vi "NEW数据采集传输系统.vi"() -> ()   [LabVIEW 2016, in "数据传输系统-04.lvlib"]
uses:
  <vilib>/Utility/miscctls.llb/LVPointTypeDef.ctl
  <vilib>/Utility/error.llb/whitespace.ctl
  <vilib>/Utility/config.llb/NI_LVConfig.lvlib
  update/update.lvlib
panel:
  in  "自动更新":bool
  in  "数据补传":bool caption="确定"
  out "数据库打开失败次数":dbl
  out "与工控通信指示灯":bool
  in  "判断数据反馈":enum16{"非严格判断", "严格判断", "不判断"}(ring)
  in  "暂停上传":bool
  in  "配置表":bool caption="确定"
  in  "updateconfiguration":T1={"主机"="27.154.58.30", "用户"="update", "密码"="std23506", "远程路径"="数据传输系统\\平台数据传输系统.exe", "下载文件名"="平台数据传输系统.exe", "软件版本"=""}
  out "标题显示":string
  in  "更新":bool
  in  "系统编码选择框":string(combo)="地表水质量监测"
  in  "数据发送通道":enum16{"TCP", "VISA"}(ring)
  in  "baud rate":u32=9600 caption="波特率"
  in  "VISA resource name":refnum<visa-resource-name> caption="VISA资源名称"
  in  "实时数据发送时间间隔/min":i32=1
  in  "数据组合发送":bool
  in  "2011发送":bool
  in  "数据发送协议":enum16{"2005-212协议", "2017-212协议"}(ring)=enum."2017-212协议"
  in  "重发时间":T2(ring)
  in  "重发日期":T3(ring)
  in  "开机启动":bool
  in  "每周自动重发":bool=TRUE
  in  "确定":bool
  in  "返回":bool
  in  "PW":string
  in  "MN":string
  in  "PORT":string
  in  "IP":string
  in  "站点设备":string
  in  "站点名称":string
  out "设置超时时间/min":i32=1
  out "状态信息":T4={"1st Error to Convert "=63, "步骤 "=enum."发送数据", "元素"="实时数据", "TCP服务端掉线计数"=0, "TCP掉线时间节点"="2019/05/08 15:24:17"} {"1st Error to Convert" items=["无错误", "参数错误", "内存已满", "超出区域", "文件结束", "文件已打开", "一般文件IO错误", "未找到文件", "文件权限错误", "磁盘已满", "路径副本", "打开过多文件", "未启用", "未找到资源文件", "无法添加资源", "未找到资源", "未找到图像", "图像内存错误", "画笔不存在", "配置错误类型", "配置未找到解析段", "配置解析错误", "配置内存错误", "错误外部代码格式", "错误外部代码偏移量", "外部代码不存在", "空窗口", "销毁窗口错误", "空菜单", "打印已中止", "错误打印记录", "打印驱动程序错误", "打印时窗口错误", "打印时内存错误", "打印对话框错误", "一般打印错误", "无效设备引用句柄", "设备未找到", "设备参数错误", "设备单位错误", "无法打开设备", "设备调用已中止", "一般错误", "用户已取消", "对象ID过低", "对象ID过高", "对象不在堆中", "未知的堆", "错误DefProc ID", "DefProc不在表格中", "范围外信息", "空方法", "未知信息", "不支持管理器调用", "错误地址", "连接过程中", "连接超时", "连接过程中", "不支持网络属性", "网络错误", "正在使用的地址", "系统缺少内存", "连接已中止", "连接已拒绝", "连接未建立", "连接已建立", "连接已关闭", "初始化错误（交互应用程序管理器）", "错误事件发生", "等待无约束事件发生处理程序", "事件发生队列溢出", "错误路径", "未发出信号量", "未识别类型（交互应用程序管理器）"]}
  out "数据接收超时指示灯":bool
  out "空闲时间/s":string
  out "系统时间":string
  out "实时小时数据上传":bool
  out "系统状态改变":bool
  out "软件版本":string
  out "掉线指示":bool
  out "核查数据上传":bool
  out "配置信息":T5
  in  "参数配置":bool
  out "反控数据发送":bool
  out "读取报文显示":string
  out "发送报文显示":string
  out "心跳包":bool
  out "通信状态":bool
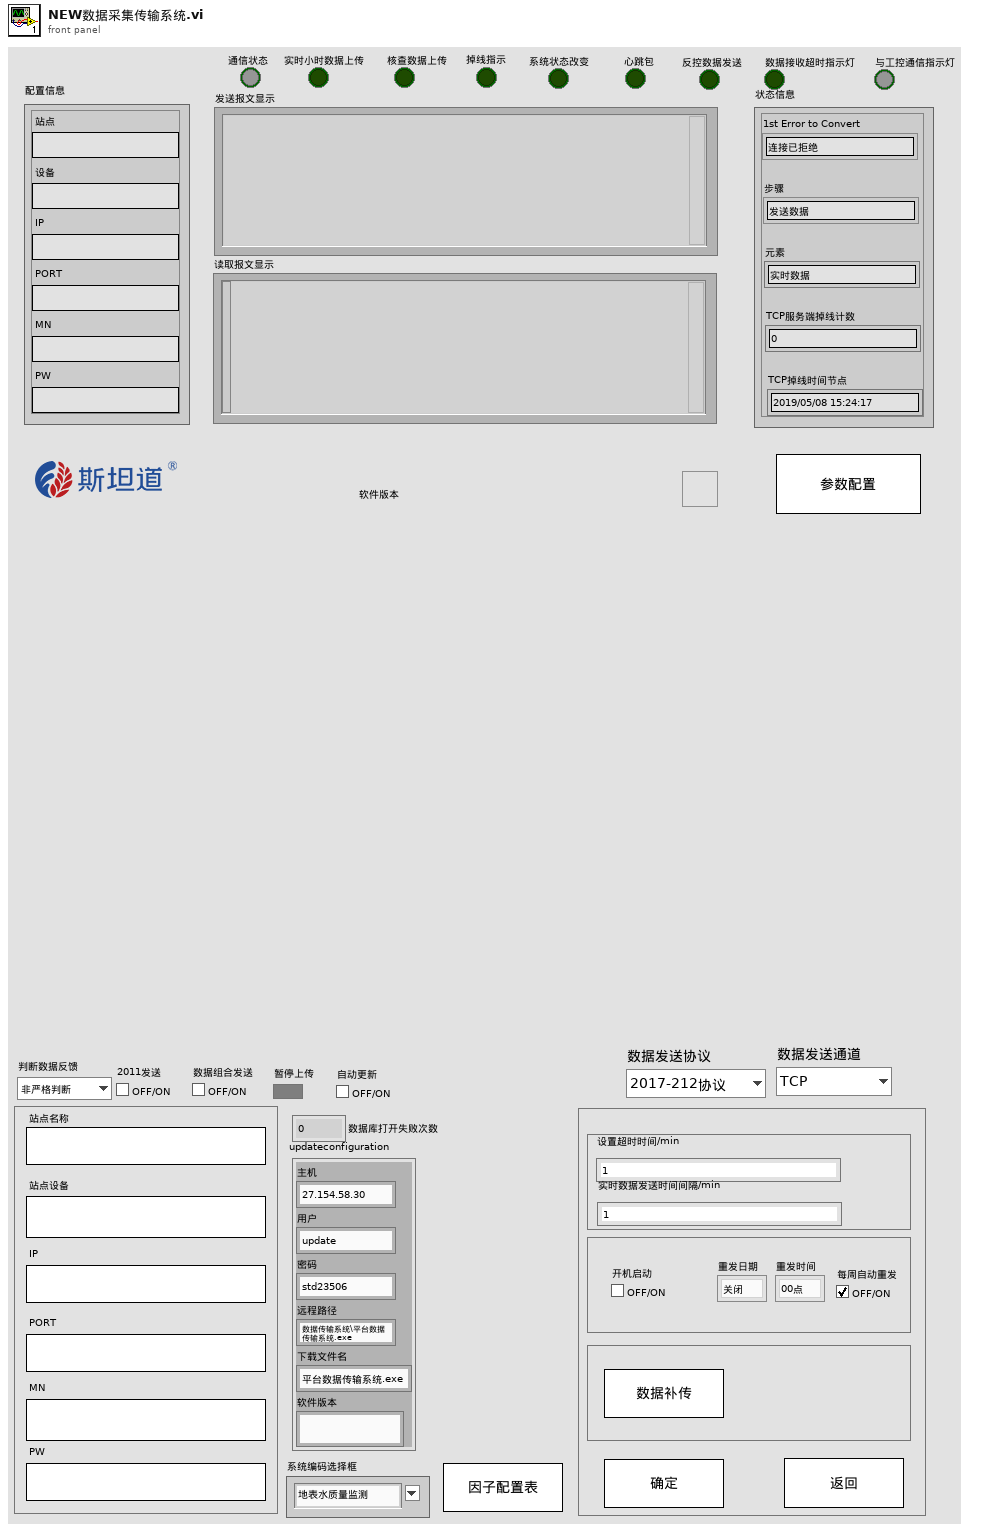
[diagram p1: front panel]
types:
  T1 = cluster{"主机":string, "用户":string, "密码":string, "远程路径":string, "下载文件名":string, "软件版本":string}
  T2 = enum16{"00点", "01点", "02点", "03点", "04点", "05点", "06点", "07点", "08点", "09点", "10点", "11点", "12点", "13点", "14点", "15点", "16点", "17点", "18点", "19点", "20点", "21点", "22点", "23点"}
  T3 = enum16{"关闭", "星期日", "星期一", "星期二", "星期三", "星期四", "星期五", "星期六"}
  T4 = cluster{"1st Error to Convert ":i32, "步骤 ":enum16{"打开连接", "发送数据", "读取数据", "数据处理", "关闭连接"}, "元素":string, "TCP服务端掉线计数":i32, "TCP掉线时间节点":string}
  T5 = cluster{"站点":string, "设备":string, "IP":string, "PORT":string, "MN":string, "PW":string}
  T6 = typedef "LVPointTypeDef.ctl" = cluster{"Horizontal":i16, "Vertical":i16}
  T7 = cluster{"setini":string, "sysini":string, "hechaini":string, "actualwrite":string, "actualread":string, "datasent":string, "反控命令信息队列":string, "反控与仪器交互":string}
  T8 = typedef "imagedata.ctl" = cluster{"image type":i32, "image depth":i32, "image":u8[], "mask":u8[], "colors":u32[], "Rectangle":cluster{"left":i16, "top":i16, "right":i16, "bottom":i16}}
  T9 = cluster{"配置表格[0]":string, "配置表格[1]":string, "配置表格[2]":string, "配置表格[3]":string, "配置表格[4]":string, "配置表格[5]":string, "配置表格[6]":string, "配置表格[7]":string, "配置表格[8]":string, "配置表格[9]":string, "配置表格[10]":string, "配置表格[11]":string, "配置表格[12]":string, "配置表格[13]":string, "配置表格[14]":string, "配置表格[15]":string, "配置表格[16]":string, "配置表格[17]":string, "配置表格[18]":string, "配置表格[19]":string, "配置表格[20]":string, "配置表格[21]":string, "配置表格[22]":string, "配置表格[23]":string, "配置表格[24]":string, "配置表格[25]":string, "配置表格[26]":string, "配置表格[27]":string, "配置表格[28]":string, "配置表格[29]":string, "配置表格[30]":string, "配置表格[31]":string, "配置表格[32]":string, "配置表格[33]":string}
  T10 = cluster{"[0]":dbl, "[1]":dbl, "[2]":dbl, "[3]":dbl, "[4]":dbl, "[5]":dbl, "[6]":dbl, "[7]":dbl, "[8]":dbl, "[9]":dbl, "[10]":dbl, "[11]":dbl, "[12]":dbl, "[13]":dbl, "[14]":dbl, "[15]":dbl, "[16]":dbl, "[17]":dbl, "[18]":dbl, "[19]":dbl, "[20]":dbl, "[21]":dbl, "[22]":dbl, "[23]":dbl, "[24]":dbl, "[25]":dbl, "[26]":dbl, "[27]":dbl, "[28]":dbl, "[29]":dbl, "[30]":dbl, "[31]":dbl, "[32]":dbl, "[33]":dbl}
  T11 = cluster{"host":string, "port":u16, "user":string, "password":string, "远端地址":string}
  T12 = typedef "NI_LVConfig.lvlib/Config Data RefNum.ctl" = refnum<k1>
  T13 = cluster{"[0]":string, "[1]":string, "[2]":string, "[3]":string, "[4]":string, "[5]":string}
  T14 = cluster{"[0]":string, "[1]":string, "[2]":string, "[3]":string, "[4]":string, "[5]":string, "[6]":string, "[7]":string}
  T15 = cluster{"[0]":string, "[1]":string, "[2]":string, "[3]":string, "[4]":string}
  T16 = cluster{"[0]":string, "[1]":string, "[2]":string, "[3]":string, "[4]":string, "[5]":string, "[6]":string, "[7]":string, "[8]":string, "[9]":string, "[10]":string, "[11]":string, "[12]":string, "[13]":string, "[14]":string}
  T17 = cluster{"[0]":string, "[1]":string, "[2]":string, "[3]":string, "[4]":string, "[5]":string, "[6]":string, "[7]":string, "[8]":string, "[9]":string, "[10]":string, "[11]":string, "[12]":string, "[13]":string, "[14]":string, "[15]":string, "[16]":string, "[17]":string, "[18]":string, "[19]":string, "[20]":string, "[21]":string, "[22]":string, "[23]":string, "[24]":string, "[25]":string, "[26]":string, "[27]":string, "[28]":string, "[29]":string, "[30]":string, "[31]":string, "[32]":string, "[33]":string}
  T18 = cluster{"[0]":string, "[1]":string, "[2]":string, "[3]":string, "[4]":string, "[5]":string, "[6]":string, "[7]":string, "[8]":string, "[9]":string, "[10]":string, "[11]":string, "[12]":string}
  T19 = typedef "whitespace.ctl" = u16
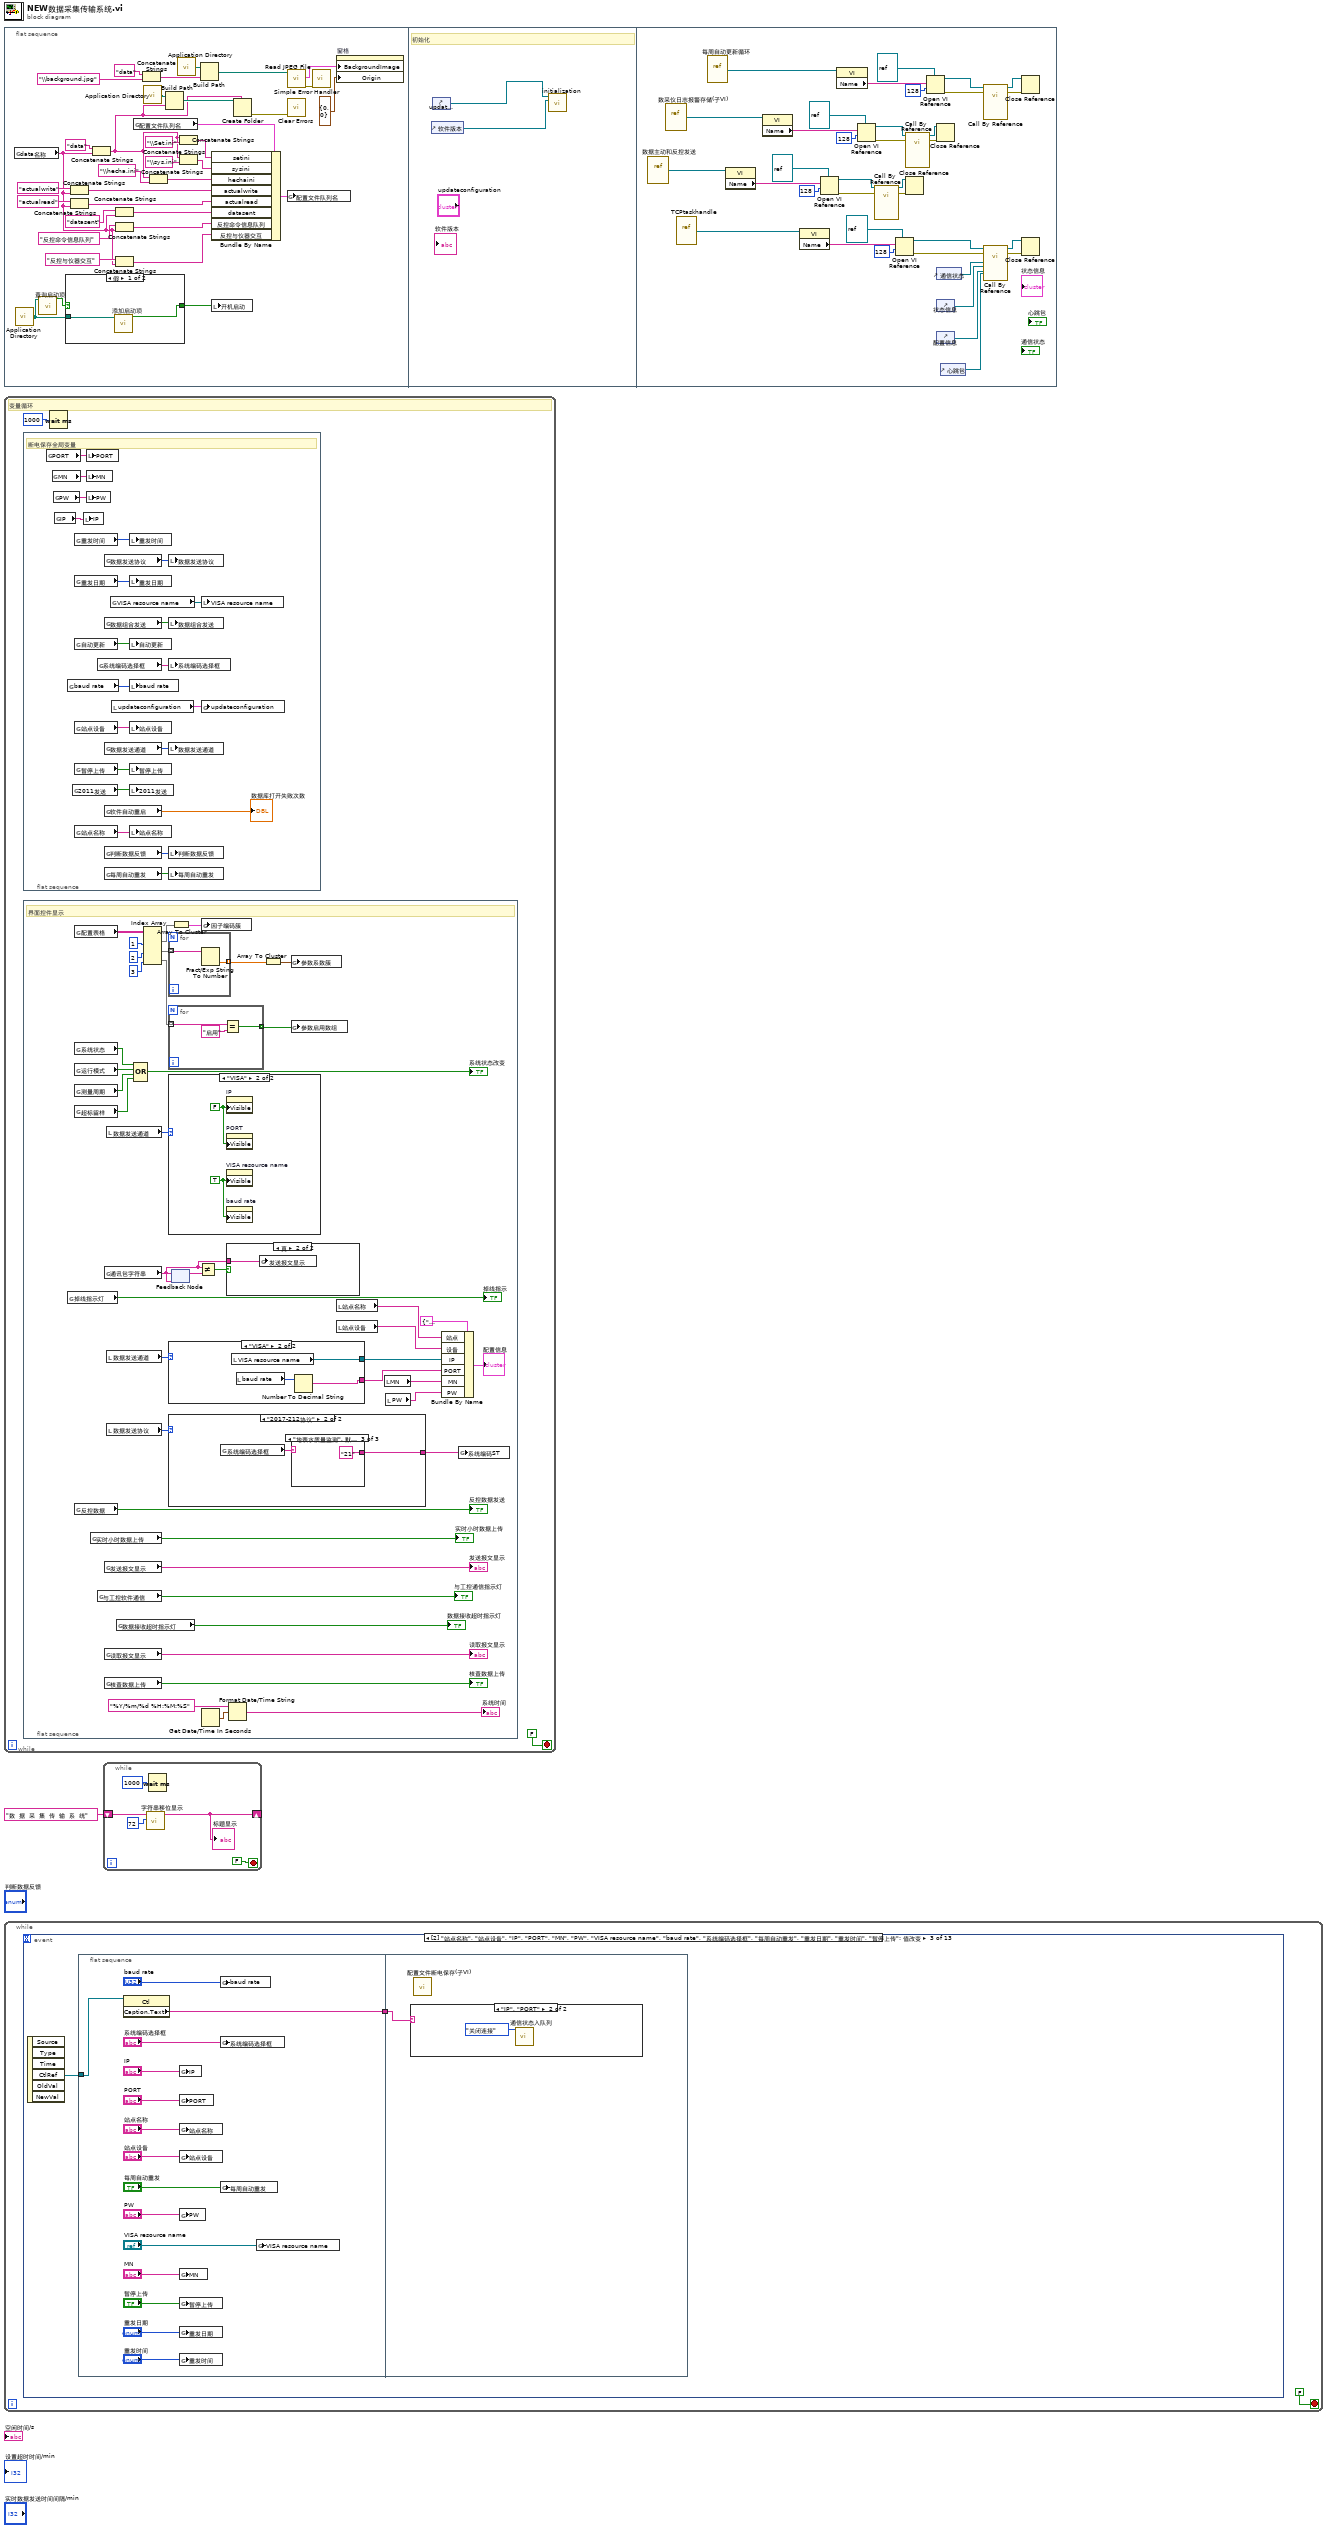
[diagram p0: block diagram]
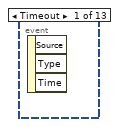
[diagram p2: hidden frame]
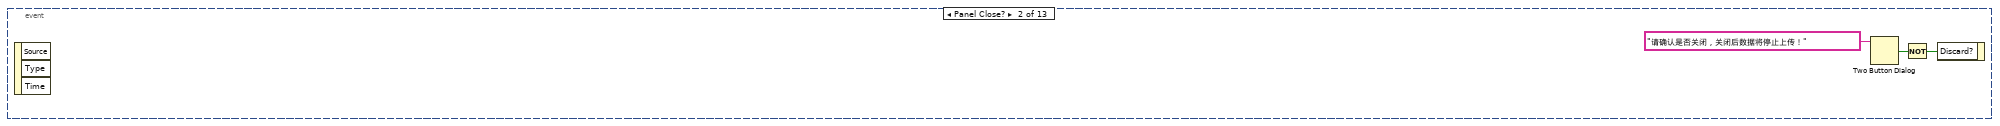
[diagram p3: hidden frame]
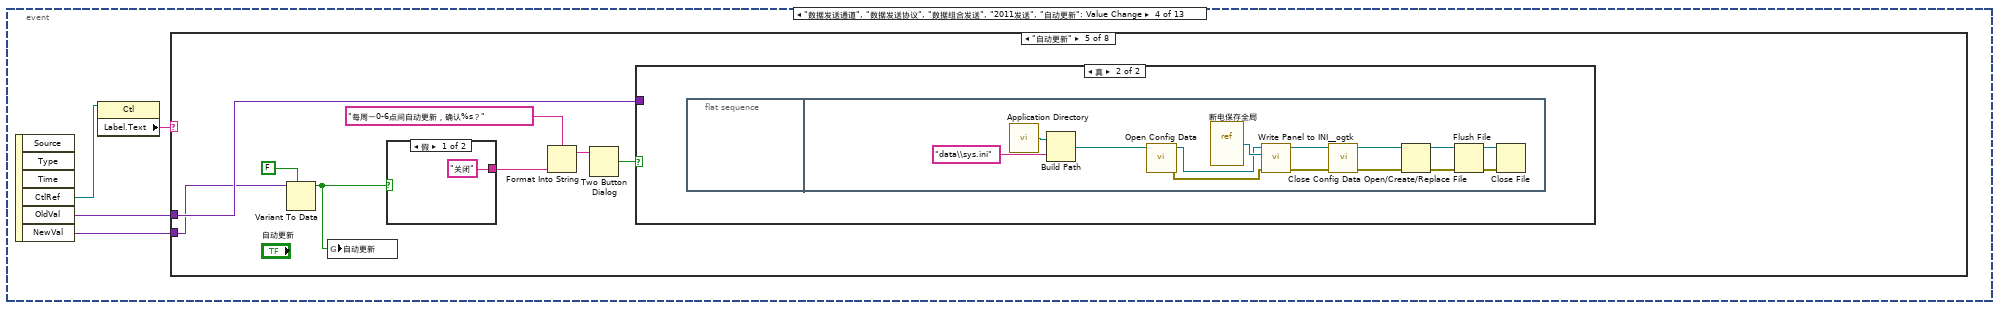
[diagram p5: hidden frame]
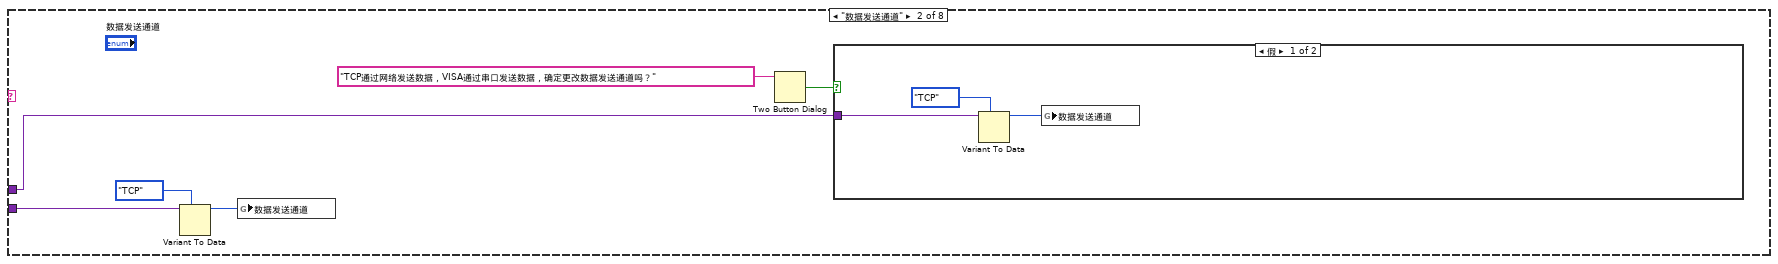
[diagram p7: hidden frame]
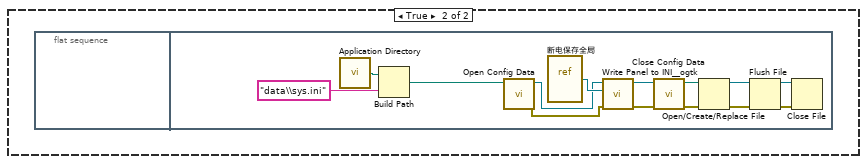
[diagram p8: hidden frame]
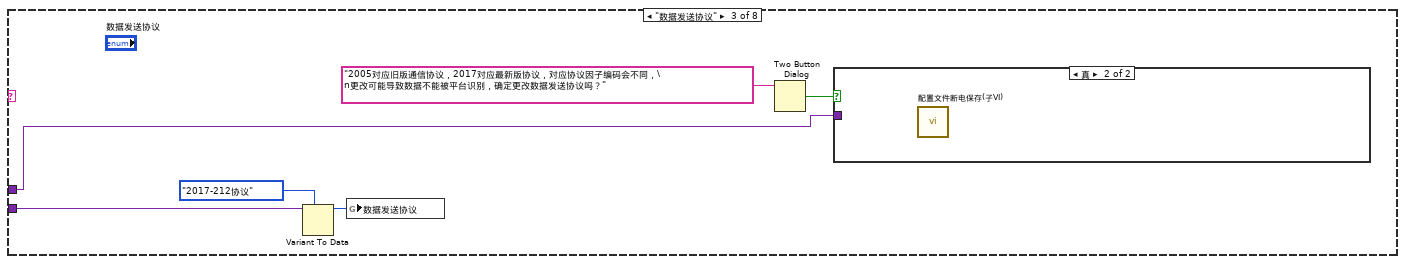
[diagram p9: hidden frame]
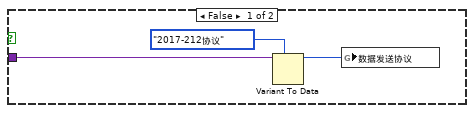
[diagram p10: hidden frame]
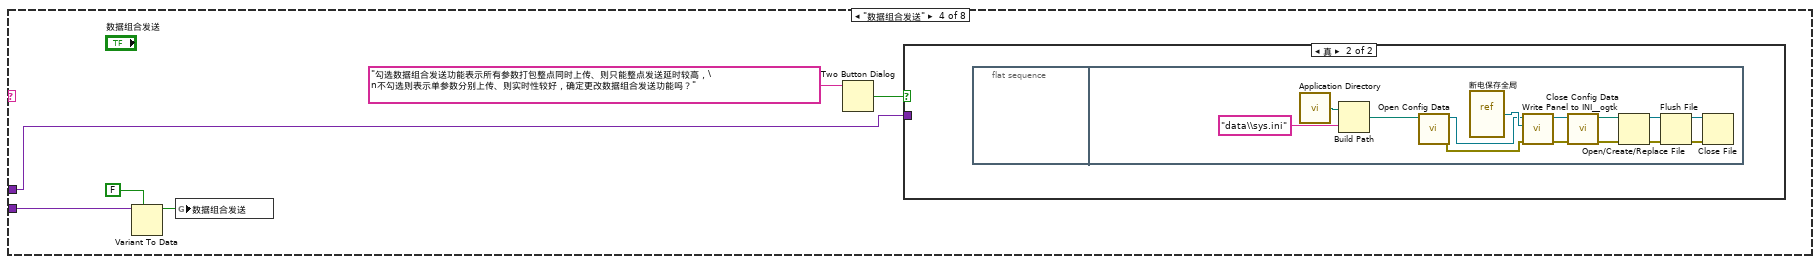
[diagram p11: hidden frame]
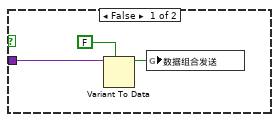
[diagram p12: hidden frame]
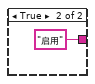
[diagram p13: hidden frame]
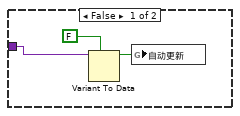
[diagram p14: hidden frame]
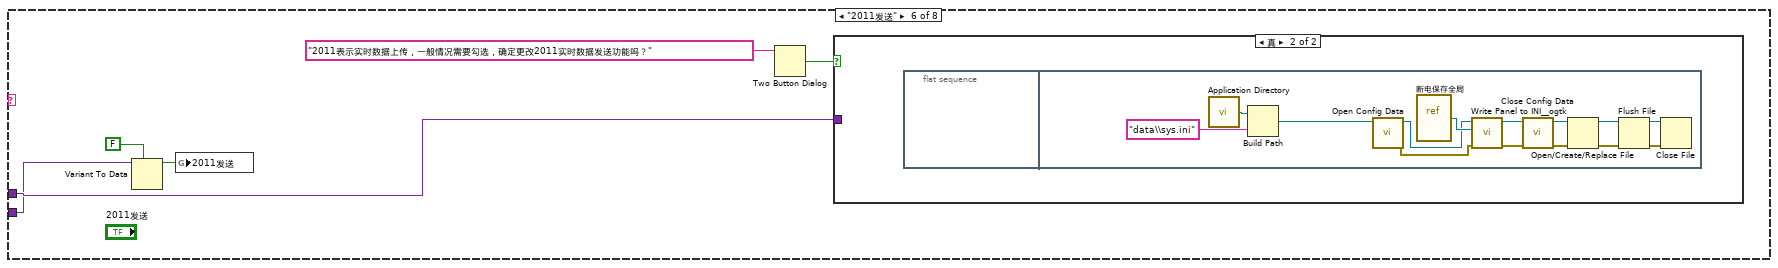
[diagram p15: hidden frame]
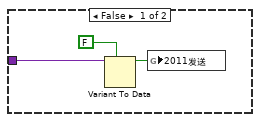
[diagram p16: hidden frame]
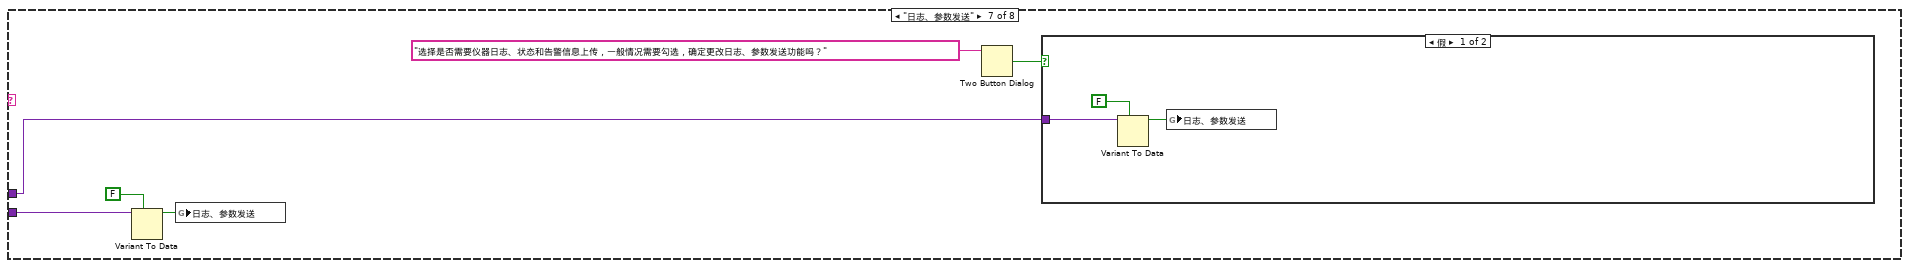
[diagram p17: hidden frame]
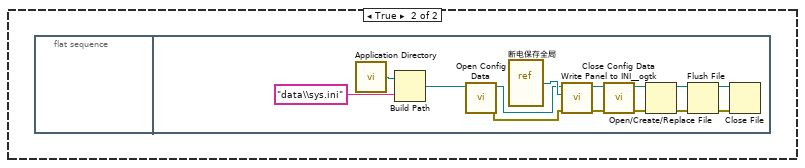
[diagram p18: hidden frame]
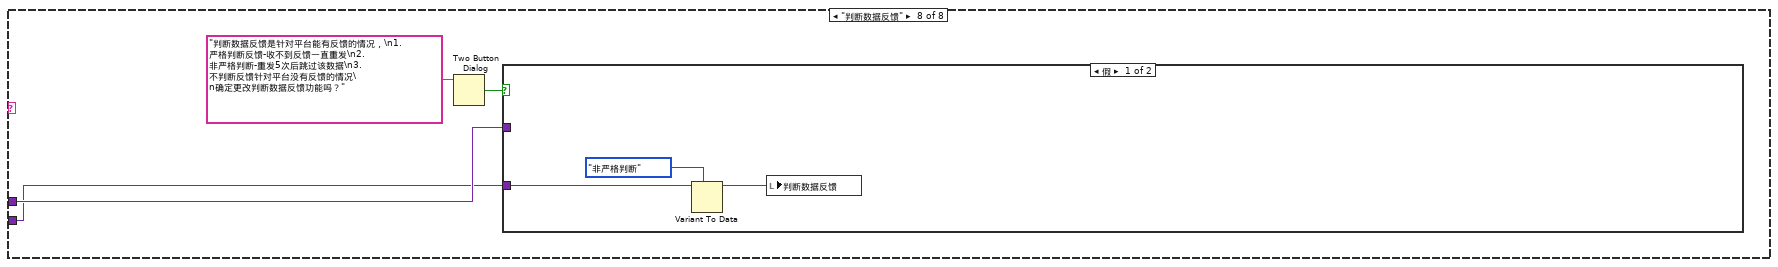
[diagram p19: hidden frame]
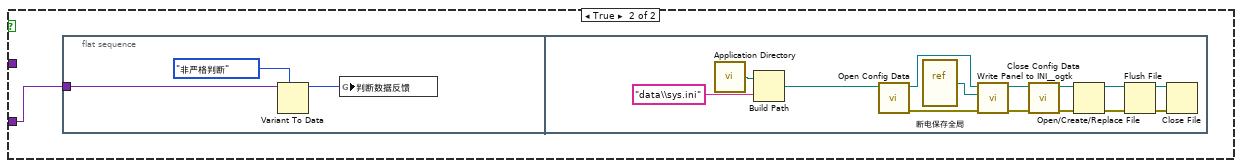
[diagram p20: hidden frame]
diagram:
  n1 = flat-sequence {
    frame #0 {
      n2 = global read "断电保存全局.vi" "data名称"() -> (w15:string)
      n3 = call <vilib>:"Application Directory.vi"() -> ("Application Directory"=w4:path)
      n4 = call "查询启动项.vi"("启动文件路径"=w4) -> ("包含启动项"=w3:bool)  [unwired: 9 in, 1 out]
      n5 = case shown="假" w3 {
        selector: w3 -> [_ w39]
        tunnel: w4 -> [w38 _]
        tunnel: [w37 w39] -> w2
        frame False {
          n6 = call "添加启动项.vi"("启动文件路径"=w38) -> ("添加成功标记"=w37:bool)  [unwired: 9 in, 1 out]
        }
        frame True {
        }
      }
      n7 = Concatenate Strings("actualwrite" ("名称（未命名）"), w15) -> (w24:string)
      n8 = Concatenate Strings("actualread" ("名称（未命名）"), w15) -> (w22:string)
      n9 = Concatenate Strings("data" ("对话框窗口（创建文件夹）"), w15) -> (w29:string)
      n10 = Concatenate Strings("datasent" ("名称（未命名）"), w15) -> (w20:string)
      n11 = Concatenate Strings("反控命令信息队列" ("名称（未命名）"), w15) -> (w13:string)
      n12 = Concatenate Strings("反控与仪器交互" ("名称（未命名）"), w15) -> (w14:string)
      n13 = global read "断电保存全局.vi" "配置文件队列名"() -> (w19:T7)
      n14 = Concatenate Strings("data" ("名称或相对路径"), "\\background.jpg" ("名称或相对路径")) -> (w10:string)
      n15 = call <vilib>:"Application Directory.vi"() -> ("Application Directory"=w35:path)
      n16 = Concatenate Strings(w29, "\\hecha.ini" ("名称或相对路径")) -> (w27:string)
      n17 = Build Path(base path=w35, name or relative path=w29) -> (appended path=w34:path)
      n18 = call <vilib>:"Application Directory.vi"() -> ("Application Directory"=w5:path)
      n19 = Concatenate Strings(w29, "\\Set.ini" ("名称或相对路径")) -> (w31:string)
      n20 = Concatenate Strings(w29, "\\sys.ini" ("名称或相对路径")) -> (w28:string)
      n21 = Build Path(base path=w5, name or relative path=w10) -> (appended path=w6:path)
      n22 = Bundle By Name(cluster=w19, "setini"=w31, "sysini"=w28, "hechaini"=w27, "actualwrite"=w24, "actualread"=w22, "datasent"=w20, "反控命令信息队列"=w13, "反控与仪器交互"=w14) -> (w18:T7)
      n23 = local write "开机启动"(w2) -> ()
      n24 = Create Folder(prompt (Create Folder)=w29, path (use dialog)=w34) -> (error out=w33:errorcluster)  [unwired: 1 in, 2 out]
      n25 = call <vilib>:"Read JPEG File.vi"("path to JPEG file"=w6) -> ("error out"=w8:errorcluster, "image data"=w7:T8)  [unwired: 8 in, 1 out]
      n26 = call <vilib>:"Clear Errors.vi"("error in (no error)"=w33) -> ()  [unwired: 5 in, 2 out]
      n27 = global write "断电保存全局.vi" "配置文件队列名"(w18) -> ()
      n28 = call <vilib>:"Simple Error Handler.vi"("error in (no error)"=w8) -> ()  [unwired: 4 in, 5 out]
      n29 = property on="窗格" class="Pane"("BackgroundImage"=w7, "Origin"=T6 {"Horizontal"=0, "Vertical"=0} ("原点")) -> ()  [unwired: 2 in, 2 out]
    }
    frame #1 {
      # "初始化"
      n30 = control-ref of="软件版本"() -> (w40:refnum<vi>)
      n31 = control-ref of="updateconfiguration"() -> (w41:refnum<vi>)
      n32 = call "initialization.vi"("软件版本"=w40, "updateconfiguration"=w41) -> ()  [unwired: 9 in]
    }
    frame #2 {
      n33 = vi-ref "数据主动和反控发送.vi"() -> (w69:refnum<vi>)
      n34 = vi-ref "数采仪日志报警存储(子VI).vi"() -> (w70:refnum<vi>)
      n35 = vi-ref "TCPtaskhandle.vi"() -> (w46:refnum<vi>)
      n36 = vi-ref "每周自动更新循环.vi"() -> (w61:refnum<vi>)
      n37 = property class="VI"(reference=w69) -> ("Name"=w68:string)  [unwired: 1 in, 2 out]
      n38 = property class="VI"(reference=w70) -> ("Name"=w77:string)  [unwired: 1 in, 2 out]
      n39 = property class="VI"(reference=w46) -> ("Name"=w53:string)  [unwired: 1 in, 2 out]
      n40 = Open VI Reference(type specifier VI Refnum (for type only)=refnum<vi> refnum, vi path=w68, options=128 ("选项")) -> (vi reference=w66:refnum<vi>, error out=w64:errorcluster)  [unwired: 3 in]
      n41 = property class="VI"(reference=w61) -> ("Name"=w54:string)  [unwired: 1 in, 2 out]
      n42 = Open VI Reference(type specifier VI Refnum (for type only)=refnum<vi> refnum, vi path=w77, options=128 ("选项")) -> (vi reference=w75:refnum<vi>, error out=w73:errorcluster)  [unwired: 3 in]
      n43 = call-by-ref "?"(reference=w66, error in=w64) -> (reference out=w62:refnum<vi>, error out=w63:errorcluster)  [unwired: 12 in]
      n44 = Open VI Reference(type specifier VI Refnum (for type only)=refnum<vi> refnum, vi path=w53, options=128 ("选项")) -> (vi reference=w51:refnum<vi>, error out=w49:errorcluster)  [unwired: 3 in]
      n45 = call-by-ref "?"(reference=w75, error in=w73) -> (reference out=w71:refnum<vi>, error out=w72:errorcluster)  [unwired: 12 in]
      n46 = Close Reference(reference=w62, error in (no error)=w63) -> ()  [unwired: 1 out]
      n47 = Open VI Reference(type specifier VI Refnum (for type only)=refnum<vi> refnum, vi path=w54, options=128 ("选项")) -> (vi reference=w56:refnum<vi>, error out=w58:errorcluster)  [unwired: 3 in]
      n48 = Close Reference(reference=w71, error in (no error)=w72) -> ()  [unwired: 1 out]
      n49 = control-ref of="通信状态"() -> (w45:refnum<vi>)
      n50 = control-ref of="状态信息"() -> (w44:refnum<vi>)
      n51 = control-ref of="配置信息"() -> (w43:refnum<vi>)
      n52 = control-ref of="心跳包"() -> (w42:refnum<vi>)
      n53 = call-by-ref "?"(reference=w56, error in=w58) -> (reference out=w60:refnum<vi>, error out=w59:errorcluster)  [unwired: 12 in]
      n54 = call-by-ref "?"(reference=w51, error in=w49, "心跳包"=w42, "配置信息"=w43, "状态信息"=w44, "通信状态"=w45) -> (reference out=w47:refnum<vi>, error out=w48:errorcluster)  [unwired: 8 in]
      n55 = Close Reference(reference=w60, error in (no error)=w59) -> ()  [unwired: 1 out]
      n56 = Close Reference(reference=w47, error in (no error)=w48) -> ()  [unwired: 1 out]
    }
  }
  n57 = while {
    stop <- FALSE stop-if-true
    # "变量循环"
    n58 = flat-sequence {
      frame #0 {
        # "断电保存全局变量"
        n59 = global read "断电保存全局.vi" "PORT"() -> (w164:string)
        n60 = global read "断电保存全局.vi" "MN"() -> (w163:string)
        n61 = global read "断电保存全局.vi" "PW"() -> (w162:string)
        n62 = global read "断电保存全局.vi" "IP"() -> (w165:string)
        n63 = global read "断电保存全局.vi" "baud rate"() -> (w160:u32)
        n64 = global read "断电保存全局.vi" "2011发送"() -> (w156:bool)
        n65 = global read "断电保存全局.vi" "重发时间"() -> (w151:T2)
        n66 = global read "断电保存全局.vi" "重发日期"() -> (w158:T3)
        n67 = global read "断电保存全局.vi" "自动更新"() -> (w147:bool)
        n68 = global read "断电保存全局.vi" "站点设备"() -> (w166:string)
        n69 = global read "断电保存全局.vi" "暂停上传"() -> (w149:bool)
        n70 = global read "断电保存全局.vi" "站点名称"() -> (w167:string)
        n71 = local write "IP"(w165) -> ()
        n72 = local write "PORT"(w164) -> ()
        n73 = local write "MN"(w163) -> ()
        n74 = local write "PW"(w162) -> ()
        n75 = global read "断电保存全局.vi" "系统编码选择框"() -> (w152:string)
        n76 = global read "断电保存全局.vi" "数据发送协议"() -> (w154:enum16{"2005-212协议", "2017-212协议"})
        n77 = global read "断电保存全局.vi" "数据组合发送"() -> (w155:bool)
        n78 = global read "断电保存全局.vi" "数据发送通道"() -> (w153:enum16{"TCP", "VISA"})
        n79 = global read "全局1.vi" "软件自动重启"() -> (→"数据库打开失败次数":dbl)
        n80 = global read "断电保存全局.vi" "判断数据反馈"() -> (w157:enum16{"非严格判断", "严格判断", "不判断"})
        n81 = global read "断电保存全局.vi" "每周自动重发"() -> (w159:bool)
        n82 = global read "断电保存全局.vi" "VISA resource name"() -> (w161:refnum<visa-resource-name>)
        n83 = local read "updateconfiguration"() -> (w150:T1)
        n84 = local write "重发时间"(w151) -> ()
        n85 = local write "重发日期"(w158) -> ()
        n86 = local write "自动更新"(w147) -> ()
        n87 = local write "baud rate"(w160) -> ()
        n88 = local write "站点设备"(w166) -> ()
        n89 = local write "暂停上传"(w149) -> ()
        n90 = local write "2011发送"(w156) -> ()
        n91 = local write "站点名称"(w167) -> ()
        n92 = local write "数据发送协议"(w154) -> ()
        n93 = local write "数据组合发送"(w155) -> ()
        n94 = local write "系统编码选择框"(w152) -> ()
        n95 = local write "数据发送通道"(w153) -> ()
        n96 = local write "判断数据反馈"(w157) -> ()
        n97 = local write "每周自动重发"(w159) -> ()
        n98 = local write "VISA resource name"(w161) -> ()
        n99 = global write "update全局.vi" "updateconfiguration"(w150) -> ()
      }
    }
    n100 = flat-sequence {
      frame #0 {
        # "界面控件显示"
        n101 = global read "全局 数据发送重叠.vi" "掉线指示灯"() -> (→"掉线指示":bool)
        n102 = global read "断电保存全局.vi" "配置表格"() -> (w90:string[][])
        n103 = global read "全局1.vi" "系统状态"() -> (w92:bool)
        n104 = global read "全局1.vi" "运行模式"() -> (w93:bool)
        n105 = global read "全局1.vi" "测量周期"() -> (w94:bool)
        n106 = global read "全局1.vi" "超标留样"() -> (w95:bool)
        n107 = global read "全局1.vi" "反控数据"() -> (→"反控数据发送":bool)
        n108 = global read "全局1.vi" "实时小时数据上传"() -> (→"实时小时数据上传":bool)
        n109 = global read "全局1.vi" "与工控软件通信"() -> (→"与工控通信指示灯":bool)
        n110 = global read "全局1.vi" "通讯包字符串"() -> (w102:string)
        n111 = global read "全局1.vi" "发送报文显示"() -> (→"发送报文显示":string)
        n112 = global read "全局1.vi" "读取报文显示"() -> (→"读取报文显示":string)
        n113 = global read "全局1.vi" "核查数据上传"() -> (→"核查数据上传":bool)
        n114 = local read "数据发送通道"() -> (w100:enum16{"TCP", "VISA"})
        n115 = local read "数据发送通道"() -> (w121:enum16{"TCP", "VISA"})
        n116 = local read "数据发送协议"() -> (w110:enum16{"2005-212协议", "2017-212协议"})
        n117 = global read "全局 数据发送重叠.vi" "数据接收超时指示灯"() -> (→"数据接收超时指示灯":bool)
        n118 = Compound Arithmetic op=OR ("复合运算")(w92, w93, w94, w95) -> (→"系统状态改变":bool)
        n119 = Index Array(array=w90, index (col) #1=1 ("禁用的索引 (列)"), index (col) #2=2 ("索引 (列)"), index (col) #3=3 ("索引 (列)")) -> (element #1=w88:string[], element #2=w82:string[], element #3=w84:string[])  [unwired: 3 in]
        n120 = for {
          tunnel: w82 -> [w123] mode=indexing
          tunnel: [w122] -> w81 mode=indexing
          n121 = Fract/Exp String To Number(string=w123) -> (number=w122:dbl)  [unwired: 3 in, 1 out]
        }
        n122 = for {
          tunnel: w84 -> [w126] mode=indexing
          tunnel: [w124] -> w83 mode=indexing
          n123 = Equal?(x=w126, y="启用") -> (x = y?=w124:bool)
        }
        n124 = case shown="\"VISA\"" w100 {
          frame "TCP", Default {
            w127 = TRUE ("可见")
            w128 = FALSE ("可见")
            n125 = property on="IP" class="Str"("Visible"=w127) -> ()  [unwired: 2 in, 2 out]
            n126 = property on="PORT" class="Str"("Visible"=w127) -> ()  [unwired: 2 in, 2 out]
            n127 = property on="VISA resource name" class="VISAName"("Visible"=w128) -> ()  [unwired: 2 in, 2 out]
            n128 = property on="baud rate" class="DigNum (严格)"("Visible"=w128) -> ()  [unwired: 2 in, 2 out]
          }
          frame "VISA" {
            w129 = FALSE ("可见")
            w130 = TRUE ("可见")
            n129 = property on="IP" class="Str"("Visible"=w129) -> ()  [unwired: 2 in, 2 out]
            n130 = property on="PORT" class="Str"("Visible"=w129) -> ()  [unwired: 2 in, 2 out]
            n131 = property on="VISA resource name" class="VISAName"("Visible"=w130) -> ()  [unwired: 2 in, 2 out]
            n132 = property on="baud rate" class="DigNum (严格)"("Visible"=w130) -> ()  [unwired: 2 in, 2 out]
          }
        }
        n133 = case shown="\"VISA\"" w121 {
          tunnel: [w143 w146] -> w118
          tunnel: [w142 w144] -> w115
          frame "TCP", Default {
            n134 = local read "PORT"() -> (w142:string)
            n135 = local read "IP"() -> (w143:string)
          }
          frame "VISA" {
            n136 = local read "VISA resource name"() -> (w146:refnum<visa-resource-name>)
            n137 = local read "baud rate"() -> (w145:u32)
            n138 = Number To Decimal String(number=w145) -> (decimal integer string=w144:string)  [unwired: 1 in]
          }
        }
        n139 = case shown="\"2017-212协议\"" w110 {
          tunnel: [w132 w137] -> w109
          frame "2005-212协议", Default {
            n140 = global read "断电保存全局.vi" "系统编码选择框"() -> (w133:string)
            n141 = case shown="\"地表水体污染源\"" w133 {
              tunnel: ["52" ("设备编码MN") "32" ("设备编码MN") "21" ("设备编码MN")] -> w132
              frame "污水排放过程监测" {
              }
              frame "地表水体污染源" {
              }
              frame "地表水质量监测", Default {
              }
            }
          }
          frame "2017-212协议" {
            n142 = global read "断电保存全局.vi" "系统编码选择框"() -> (w138:string)
            n143 = case shown="\"地表水质量监测\", 默认" w138 {
              tunnel: ["52" ("设备编码MN") "32" ("设备编码MN") "21" ("设备编码MN")] -> w137
              frame "污水排放过程监测" {
              }
              frame "地表水体污染源" {
              }
              frame "地表水质量监测", Default {
              }
            }
          }
        }
        n144 = feedback #1(w102) -> (w103:string)
        n145 = feedback-in #1(w102) -> ()
        n146 = Array To Cluster(array=w88) -> (cluster=w91:T9)
        n147 = Not Equal?(x=w102, y=w103) -> (x != y?=w101:bool)
        n148 = global write "断电保存全局.vi" "因子编码簇"(w91) -> ()
        n149 = Get Date/Time In Seconds() -> (seconds since 1Jan1904=w111:timestamp)
        n150 = case shown="真" w101 {
          tunnel: w102 -> [_ w131]
          frame False {
          }
          frame True {
            n151 = global write "全局1.vi" "发送报文显示"(w131) -> ()
          }
        }
        n152 = Format Date/Time String(time format string (%c)="%Y/%m/%d %H:%M:%S" ("时间格式字符串(%c)"), seconds (now)=w111) -> (date/time string=→"系统时间":string)  [unwired: 1 in]
        n153 = Array To Cluster(array=w81) -> (cluster=w85:T10)
        n154 = global write "断电保存全局.vi" "参数系数簇"(w85) -> ()
        n155 = global write "断电保存全局.vi" "参数启用数组"(w83) -> ()
        n156 = local read "站点名称"() -> (w117:string)
        n157 = local read "站点设备"() -> (w116:string)
        n158 = local read "MN"() -> (w114:string)
        n159 = local read "PW"() -> (w113:string)
        n160 = Bundle By Name(cluster=T5 {"站点"="", "设备"="", "IP"="", "PORT"="", "MN"="", "PW"=""} ("配置信息"), "站点"=w117, "设备"=w116, "IP"=w118, "PORT"=w115, "MN"=w114, "PW"=w113) -> (→"配置信息":T5)
        n161 = global write "全局1.vi" "系统编码ST"(w109) -> ()
      }
    }
    n162 = Wait (ms)(milliseconds to wait=u32 1000 ("等待时间（毫秒）")) -> ()  [unwired: 1 out]
  }
  n163 = while {
    stop <- FALSE stop-if-true
    n164 = event shown="[2] \"站点名称\", \"站点设备\", \"IP\", \"PORT\", \"MN\", \"PW\", \"VISA resource name\", \"baud rate\", \"系统编码选择框\", \"每周自动重发\", \"重发日期\", \"重发时间\", \"暂停上传\": 值改变" {
      selector: _ -> [_ _ _ _ _ _ _ _ _ _ _ _ _]
      dyn-events: _ -> [_ _ _ _ _ _ _ _ _ _ _ _ _]
      timeout: _ -> [_ _ _ _ _ _ _ _ _ _ _ _ _]
      event Timeout {
        n165 = event-data() -> ()  [unwired: 1 in, 3 out]
      }
      event Panel Close? {
        n166 = event-data() -> ()  [unwired: 1 in, 3 out]
        n167 = Two Button Dialog(message="请确认是否关闭，关闭后数据将停止上传！" ("消息")) -> (T button?=w171:bool)  [unwired: 2 in]
        n168 = Not(x=w171) -> (.not. x?=w170:bool)
        n169 = event-data("Discard?"=w170) -> ()  [unwired: 1 in, 1 out]
      }
      event "站点名称", "站点设备", "IP", "PORT", "MN", "PW", "VISA resource name", "baud rate", "系统编码选择框", "每周自动重发", "重发日期", "重发时间", "暂停上传": Value Change {
        n170 = event-data() -> ("CtlRef"=w173:refnum<vi>)  [unwired: 1 in, 5 out]
        n171 = flat-sequence {
          tunnel: w173 -> [w175]
          tunnel: [w174] -> w172
          tunnel: w172 -> [w189]
          frame #0 {
            n172 = property class="Ctl"(reference=w175) -> ("Caption.Text"=w174:string)  [unwired: 1 in, 2 out]
            n173 = global write "断电保存全局.vi" "IP"("IP") -> ()
            n174 = global write "断电保存全局.vi" "PORT"("PORT") -> ()
            n175 = global write "断电保存全局.vi" "站点名称"("站点名称") -> ()
            n176 = global write "断电保存全局.vi" "站点设备"("站点设备") -> ()
            n177 = global write "断电保存全局.vi" "PW"("PW") -> ()
            n178 = global write "断电保存全局.vi" "MN"("MN") -> ()
            n179 = global write "断电保存全局.vi" "暂停上传"("暂停上传") -> ()
            n180 = global write "断电保存全局.vi" "重发日期"("重发日期") -> ()
            n181 = global write "断电保存全局.vi" "重发时间"("重发时间") -> ()
            n182 = global write "断电保存全局.vi" "baud rate"("baud rate") -> ()
            n183 = global write "断电保存全局.vi" "系统编码选择框"("系统编码选择框") -> ()
            n184 = global write "断电保存全局.vi" "每周自动重发"("每周自动重发") -> ()
            n185 = global write "断电保存全局.vi" "VISA resource name"("VISA resource name") -> ()
          }
          frame #1 {
            n186 = case shown="\"IP\", \"PORT\"" w189 {
              frame "假", Default {
              }
              frame "IP", "PORT" {
                n187 = call "通信状态入队列.vi"("枚举"=enum16{"打开连接", "发送数据", "读取数据", "数据处理", "关闭连接"}."关闭连接") -> ()  [unwired: 10 in, 1 out]
              }
            }
            n188 = call "配置文件断电保存(子VI).vi"() -> ()  [unwired: 12 in]
          }
        }
      }
      event "数据发送通道", "数据发送协议", "数据组合发送", "2011发送", "自动更新": Value Change {
        n189 = event-data() -> ("CtlRef"=w194:refnum<vi>, "OldVal"=w192:variant, "NewVal"=w191:variant)  [unwired: 1 in, 3 out]
        n190 = property class="Ctl"(reference=w194) -> ("Label.Text"=w193:string)  [unwired: 1 in, 2 out]
        n191 = case shown="\"自动更新\"" w193 {
          tunnel: w192 -> [_ w198 w221 w230 w256 w280 w303 w324]
          tunnel: w191 -> [_ w195 w218 w227 w254 w277 w300 w323]
          frame "假", Default {
          }
          frame "数据发送通道" {
            n192 = Variant To Data(type=enum16{"TCP", "VISA"}."TCP" ("数据发送通道"), Variant=w195) -> (data=w196:enum16{"TCP", "VISA"})  [unwired: 1 in, 1 out]
            n193 = global write "断电保存全局.vi" "数据发送通道"(w196) -> ()
            n194 = Two Button Dialog(message="TCP通过网络发送数据，VISA通过串口发送数据，确定更改数据发送通道吗？" ("消息")) -> (T button?=w199:bool)  [unwired: 2 in]
            n195 = case shown="假" w199 {
              tunnel: w198 -> [w202 _]
              frame False {
                n196 = Variant To Data(type=enum16{"TCP", "VISA"}."TCP" ("数据发送通道"), Variant=w202) -> (data=w201:enum16{"TCP", "VISA"})  [unwired: 1 in, 1 out]
                n197 = global write "断电保存全局.vi" "数据发送通道"(w201) -> ()
              }
              frame True {
                n198 = flat-sequence {
                  frame #0 {
                  }
                  frame #1 {
                    n199 = call <vilib>:"Application Directory.vi"() -> ("Application Directory"=w204:path)
                    n200 = Build Path(base path=w204, name or relative path="data\\sys.ini" ("名称或相对路径")) -> (appended path=w206:path)
                    n201 = call <vilib>:"Open Config Data.vi"("configuration file path"=w206) -> ("error out"=w210:errorcluster, "refnum"=w207:T12)  [unwired: 8 in, 1 out]
                    n202 = vi-ref "断电保存全局.vi"() -> (w208:refnum<vi>)
                    n203 = call <userlib>:"Write Panel to INI__ogtk.vi"("error in (no error)"=w210, "VI ref"=w208, "refnum"=w207) -> ("error out"=w211:errorcluster, "refnum out"=w209:T12)  [unwired: 7 in]
                    n204 = call <vilib>:"Close Config Data.vi"("error in (no error)"=w211, "refnum"=w209) -> ("error out"=w216:errorcluster, "file path"=w217:path)  [unwired: 8 in]
                    n205 = Open/Create/Replace File(file path (use dialog)=w217, error in=w216) -> (refnum out=w213:refnum<file>, error out=w212:errorcluster)  [unwired: 4 in, 1 out]
                    n206 = Flush File(refnum=w213, error in=w212) -> (refnum out=w214:refnum<file>, error out=w215:errorcluster)
                    n207 = Close File(refnum=w214, error in=w215) -> ()  [unwired: 2 out]
                  }
                }
              }
            }
          }
          frame "数据发送协议" {
            n208 = Variant To Data(type=enum16{"2005-212协议", "2017-212协议"}."2017-212协议" ("数据"), Variant=w218) -> (data=w219:enum16{"2005-212协议", "2017-212协议"})  [unwired: 1 in, 1 out]
            n209 = global write "断电保存全局.vi" "数据发送协议"(w219) -> ()
            n210 = Two Button Dialog(message="2005对应旧版通信协议，2017对应最新版协议，对应协议因子编码会不同，\n更改可能导致数据不能被平台识别，确定更改数据发送协议吗？" ("消息")) -> (T button?=w222:bool)  [unwired: 2 in]
            n211 = case shown="真" w222 {
              tunnel: w221 -> [w226 _]
              frame False {
                n212 = Variant To Data(type=enum16{"2005-212协议", "2017-212协议"}."2017-212协议" ("数据"), Variant=w226) -> (data=w224:enum16{"2005-212协议", "2017-212协议"})  [unwired: 1 in, 1 out]
                n213 = global write "断电保存全局.vi" "数据发送协议"(w224) -> ()
              }
              frame True {
                n214 = call "配置文件断电保存(子VI).vi"() -> ()  [unwired: 12 in]
              }
            }
          }
          frame "数据组合发送" {
            n215 = Variant To Data(type=FALSE, Variant=w227) -> (data=w228:bool)  [unwired: 1 in, 1 out]
            n216 = global write "断电保存全局.vi" "数据组合发送"(w228) -> ()
            n217 = Two Button Dialog(message="勾选数据组合发送功能表示所有参数打包整点同时上传、则只能整点发送延时较高，\n不勾选则表示单参数分别上传、则实时性较好，确定更改数据组合发送功能吗？" ("消息")) -> (T button?=w231:bool)  [unwired: 2 in]
            n218 = case shown="真" w231 {
              tunnel: w230 -> [w234 _]
              frame False {
                n219 = Variant To Data(type=FALSE, Variant=w234) -> (data=w233:bool)  [unwired: 1 in, 1 out]
                n220 = global write "断电保存全局.vi" "数据组合发送"(w233) -> ()
              }
              frame True {
                n221 = flat-sequence {
                  frame #0 {
                  }
                  frame #1 {
                    n222 = call <vilib>:"Application Directory.vi"() -> ("Application Directory"=w236:path)
                    n223 = Build Path(base path=w236, name or relative path="data\\sys.ini" ("名称或相对路径")) -> (appended path=w238:path)
                    n224 = call <vilib>:"Open Config Data.vi"("configuration file path"=w238) -> ("error out"=w242:errorcluster, "refnum"=w239:T12)  [unwired: 8 in, 1 out]
                    n225 = vi-ref "断电保存全局.vi"() -> (w240:refnum<vi>)
                    n226 = call <userlib>:"Write Panel to INI__ogtk.vi"("error in (no error)"=w242, "VI ref"=w240, "refnum"=w239) -> ("error out"=w243:errorcluster, "refnum out"=w241:T12)  [unwired: 7 in]
                    n227 = call <vilib>:"Close Config Data.vi"("error in (no error)"=w243, "refnum"=w241) -> ("error out"=w248:errorcluster, "file path"=w249:path)  [unwired: 8 in]
                    n228 = Open/Create/Replace File(file path (use dialog)=w249, error in=w248) -> (refnum out=w245:refnum<file>, error out=w244:errorcluster)  [unwired: 4 in, 1 out]
                    n229 = Flush File(refnum=w245, error in=w244) -> (refnum out=w246:refnum<file>, error out=w247:errorcluster)
                    n230 = Close File(refnum=w246, error in=w247) -> ()  [unwired: 2 out]
                  }
                }
              }
            }
          }
          frame "自动更新" {
            n231 = Variant To Data(type=FALSE, Variant=w254) -> (data=w252:bool)  [unwired: 1 in, 1 out]
            n232 = global write "断电保存全局.vi" "自动更新"(w252) -> ()
            n233 = case shown="假" w252 {
              tunnel: ["关闭" "启用"] -> w251
              frame False {
              }
              frame True {
              }
            }
            n234 = Format Into String(format string="每周一0-6点间自动更新，确认%s？" ("消息"), w251) -> (resulting string=w250:string)  [unwired: 2 in, 1 out]
            n235 = Two Button Dialog(message=w250) -> (T button?=w257:bool)  [unwired: 2 in]
            n236 = case shown="真" w257 {
              tunnel: w256 -> [w261 _]
              frame False {
                n237 = Variant To Data(type=FALSE, Variant=w261) -> (data=w260:bool)  [unwired: 1 in, 1 out]
                n238 = global write "断电保存全局.vi" "自动更新"(w260) -> ()
              }
              frame True {
                n239 = flat-sequence {
                  frame #0 {
                  }
                  frame #1 {
                    n240 = call <vilib>:"Application Directory.vi"() -> ("Application Directory"=w263:path)
                    n241 = Build Path(base path=w263, name or relative path="data\\sys.ini" ("名称或相对路径")) -> (appended path=w265:path)
                    n242 = call <vilib>:"Open Config Data.vi"("configuration file path"=w265) -> ("error out"=w269:errorcluster, "refnum"=w266:T12)  [unwired: 8 in, 1 out]
                    n243 = vi-ref "断电保存全局.vi"() -> (w267:refnum<vi>)
                    n244 = call <userlib>:"Write Panel to INI__ogtk.vi"("error in (no error)"=w269, "VI ref"=w267, "refnum"=w266) -> ("error out"=w270:errorcluster, "refnum out"=w268:T12)  [unwired: 7 in]
                    n245 = call <vilib>:"Close Config Data.vi"("error in (no error)"=w270, "refnum"=w268) -> ("error out"=w275:errorcluster, "file path"=w276:path)  [unwired: 8 in]
                    n246 = Open/Create/Replace File(file path (use dialog)=w276, error in=w275) -> (refnum out=w272:refnum<file>, error out=w271:errorcluster)  [unwired: 4 in, 1 out]
                    n247 = Flush File(refnum=w272, error in=w271) -> (refnum out=w273:refnum<file>, error out=w274:errorcluster)
                    n248 = Close File(refnum=w273, error in=w274) -> ()  [unwired: 2 out]
                  }
                }
              }
            }
          }
          frame "2011发送" {
            n249 = Variant To Data(type=FALSE, Variant=w277) -> (data=w278:bool)  [unwired: 1 in, 1 out]
            n250 = global write "断电保存全局.vi" "2011发送"(w278) -> ()
            n251 = Two Button Dialog(message="2011表示实时数据上传，一般情况需要勾选，确定更改2011实时数据发送功能吗？" ("消息")) -> (T button?=w281:bool)  [unwired: 2 in]
            n252 = case shown="真" w281 {
              tunnel: w280 -> [w284 _]
              frame False {
                n253 = Variant To Data(type=FALSE, Variant=w284) -> (data=w283:bool)  [unwired: 1 in, 1 out]
                n254 = global write "断电保存全局.vi" "2011发送"(w283) -> ()
              }
              frame True {
                n255 = flat-sequence {
                  frame #0 {
                  }
                  frame #1 {
                    n256 = call <vilib>:"Application Directory.vi"() -> ("Application Directory"=w286:path)
                    n257 = Build Path(base path=w286, name or relative path="data\\sys.ini" ("名称或相对路径")) -> (appended path=w288:path)
                    n258 = call <vilib>:"Open Config Data.vi"("configuration file path"=w288) -> ("error out"=w292:errorcluster, "refnum"=w289:T12)  [unwired: 8 in, 1 out]
                    n259 = vi-ref "断电保存全局.vi"() -> (w290:refnum<vi>)
                    n260 = call <userlib>:"Write Panel to INI__ogtk.vi"("error in (no error)"=w292, "VI ref"=w290, "refnum"=w289) -> ("error out"=w293:errorcluster, "refnum out"=w291:T12)  [unwired: 7 in]
                    n261 = call <vilib>:"Close Config Data.vi"("error in (no error)"=w293, "refnum"=w291) -> ("error out"=w298:errorcluster, "file path"=w299:path)  [unwired: 8 in]
                    n262 = Open/Create/Replace File(file path (use dialog)=w299, error in=w298) -> (refnum out=w295:refnum<file>, error out=w294:errorcluster)  [unwired: 4 in, 1 out]
                    n263 = Flush File(refnum=w295, error in=w294) -> (refnum out=w296:refnum<file>, error out=w297:errorcluster)
                    n264 = Close File(refnum=w296, error in=w297) -> ()  [unwired: 2 out]
                  }
                }
              }
            }
          }
          frame "日志、参数发送" {
            n265 = Variant To Data(type=FALSE, Variant=w300) -> (data=w301:bool)  [unwired: 1 in, 1 out]
            n266 = global write "断电保存全局.vi" "日志、参数发送"(w301) -> ()
            n267 = Two Button Dialog(message="选择是否需要仪器日志、状态和告警信息上传，一般情况需要勾选，确定更改日志、参数发送功能吗？" ("消息")) -> (T button?=w304:bool)  [unwired: 2 in]
            n268 = case shown="假" w304 {
              tunnel: w303 -> [w307 _]
              frame False {
                n269 = Variant To Data(type=FALSE, Variant=w307) -> (data=w306:bool)  [unwired: 1 in, 1 out]
                n270 = global write "断电保存全局.vi" "日志、参数发送"(w306) -> ()
              }
              frame True {
                n271 = flat-sequence {
                  frame #0 {
                  }
                  frame #1 {
                    n272 = call <vilib>:"Application Directory.vi"() -> ("Application Directory"=w309:path)
                    n273 = Build Path(base path=w309, name or relative path="data\\sys.ini" ("名称或相对路径")) -> (appended path=w311:path)
                    n274 = call <vilib>:"Open Config Data.vi"("configuration file path"=w311) -> ("error out"=w315:errorcluster, "refnum"=w312:T12)  [unwired: 8 in, 1 out]
                    n275 = vi-ref "断电保存全局.vi"() -> (w313:refnum<vi>)
                    n276 = call <userlib>:"Write Panel to INI__ogtk.vi"("error in (no error)"=w315, "VI ref"=w313, "refnum"=w312) -> ("error out"=w316:errorcluster, "refnum out"=w314:T12)  [unwired: 7 in]
                    n277 = call <vilib>:"Close Config Data.vi"("error in (no error)"=w316, "refnum"=w314) -> ("error out"=w321:errorcluster, "file path"=w322:path)  [unwired: 8 in]
                    n278 = Open/Create/Replace File(file path (use dialog)=w322, error in=w321) -> (refnum out=w318:refnum<file>, error out=w317:errorcluster)  [unwired: 4 in, 1 out]
                    n279 = Flush File(refnum=w318, error in=w317) -> (refnum out=w319:refnum<file>, error out=w320:errorcluster)
                    n280 = Close File(refnum=w319, error in=w320) -> ()  [unwired: 2 out]
                  }
                }
              }
            }
          }
          frame "判断数据反馈" {
            n281 = Two Button Dialog(message="判断数据反馈是针对平台能有反馈的情况，\n1.严格判断反馈-收不到反馈一直重发\n2.非严格判断-重发5次后跳过该数据\n3.不判断反馈针对平台没有反馈的情况\n确定更改判断数据反馈功能吗？" ("消息")) -> (T button?=w325:bool)  [unwired: 2 in]
            n282 = case shown="假" w325 {
              tunnel: w324 -> [_ _]
              tunnel: w323 -> [w328 w330]
              frame False {
                n283 = Variant To Data(type=enum16{"非严格判断", "严格判断", "不判断"}."非严格判断" ("判断数据反馈"), Variant=w328) -> (data=w327:enum16{"非严格判断", "严格判断", "不判断"})  [unwired: 1 in, 1 out]
                n284 = local write "判断数据反馈"(w327) -> ()
              }
              frame True {
                n285 = flat-sequence {
                  tunnel: w330 -> [w331]
                  frame #0 {
                    n286 = Variant To Data(type=enum16{"非严格判断", "严格判断", "不判断"}."非严格判断" ("判断数据反馈"), Variant=w331) -> (data=w333:enum16{"非严格判断", "严格判断", "不判断"})  [unwired: 1 in, 1 out]
                    n287 = global write "断电保存全局.vi" "判断数据反馈"(w333) -> ()
                  }
                  frame #1 {
                    n288 = call <vilib>:"Application Directory.vi"() -> ("Application Directory"=w334:path)
                    n289 = Build Path(base path=w334, name or relative path="data\\sys.ini" ("名称或相对路径")) -> (appended path=w336:path)
                    n290 = call <vilib>:"Open Config Data.vi"("configuration file path"=w336) -> ("error out"=w340:errorcluster, "refnum"=w337:T12)  [unwired: 8 in, 1 out]
                    n291 = vi-ref "断电保存全局.vi"() -> (w338:refnum<vi>)
                    n292 = call <userlib>:"Write Panel to INI__ogtk.vi"("error in (no error)"=w340, "VI ref"=w338, "refnum"=w337) -> ("error out"=w341:errorcluster, "refnum out"=w339:T12)  [unwired: 7 in]
                    n293 = call <vilib>:"Close Config Data.vi"("error in (no error)"=w341, "refnum"=w339) -> ("error out"=w346:errorcluster, "file path"=w347:path)  [unwired: 8 in]
                    n294 = Open/Create/Replace File(file path (use dialog)=w347, error in=w346) -> (refnum out=w343:refnum<file>, error out=w342:errorcluster)  [unwired: 4 in, 1 out]
                    n295 = Flush File(refnum=w343, error in=w342) -> (refnum out=w344:refnum<file>, error out=w345:errorcluster)
                    n296 = Close File(refnum=w344, error in=w345) -> ()  [unwired: 2 out]
                  }
                }
              }
            }
          }
        }
      }
      event "确定": Value Change {
        n297 = event-data() -> ()  [unwired: 1 in, 6 out]
        n298 = call "通信状态入队列.vi"("枚举"=enum16{"打开连接", "发送数据", "读取数据", "数据处理", "关闭连接"}."关闭连接") -> ()  [unwired: 10 in, 1 out]
      }
      event "配置表": Value Change {
        n299 = event-data() -> ()  [unwired: 1 in, 6 out]
        n300 = call "参数配置表.vi"() -> ()  [unwired: 12 in]
      }
      event "参数配置": Value Change {
        n301 = event-data() -> ()  [unwired: 1 in, 6 out]
        n302 = property on="窗格" class="Pane"("Origin"=T6 {"Horizontal"=0, "Vertical"=1000} ("原点")) -> ()  [unwired: 2 in, 2 out]
        n303 = call <vilib>:"Application Directory.vi"() -> ("Application Directory"=w350:path)
        n304 = call "查询启动项.vi"("启动文件路径"=w350) -> ("包含启动项"=w349:bool)  [unwired: 9 in, 1 out]
        n305 = local write "开机启动"(w349) -> ()
      }
      event "返回": Value Change {
        n306 = event-data() -> ()  [unwired: 1 in, 6 out]
        n307 = property on="窗格" class="Pane"("Origin"=T6 {"Horizontal"=0, "Vertical"=0} ("原点")) -> ()  [unwired: 2 in, 2 out]
      }
      event "数据补传": Value Change {
        n308 = event-data() -> ()  [unwired: 1 in, 6 out]
        n309 = global read "全局1.vi" "数据发送起始时间"() -> (w353:timestamp)
        n310 = call "数据补传对话框.vi"("起始时间"=w353) -> ("结束时间输出"=w354:timestamp, "起始时间输出"=w355:timestamp, "输出"=w356:bool)  [unwired: 8 in]
        n311 = case shown="真" w356 {
          tunnel: w355 -> [_ w357]
          tunnel: w354 -> [_ w362]
          frame False {
          }
          frame True {
            n312 = global write "断电保存全局.vi" "数据重发结束时间"(w362) -> ()
            n313 = global write "全局1.vi" "数据发送起始时间"(w357) -> ()
            n314 = global write "断电保存全局.vi" "数据重发"(TRUE ("数据重发")) -> ()
            n315 = global read "断电保存全局.vi" "数据组合发送"() -> (w370:bool)
            n316 = Format Date/Time String(time format string (%c)="%Y/%m/%d %H:%M:%S" ("时间格式字符串(%c)"), seconds (now)=w357) -> (date/time string=w358:string)  [unwired: 1 in]
            n317 = global write "全局 水样时间.vi" "剖面多参数数据时间"(w358) -> ()
            n318 = global write "全局 水样时间.vi" "剖面数据时间"(w358) -> ()
            n319 = global write "断电保存全局.vi" "数据重发时间戳"(w358) -> ()
            n320 = case shown="假" w370 {
              tunnel: w358 -> [w372 _]
              frame False {
                n321 = global write "全局 时间2.vi" "标样核查索引起始时间"(w372) -> ()
                n322 = global write "全局 时间2.vi" "加标回收索引起始时间"(w372) -> ()
                n323 = global write "全局 时间2.vi" "跨度核查索引起始时间"(w372) -> ()
                n324 = global write "全局 时间2.vi" "零点核查索引起始时间"(w372) -> ()
                n325 = Initialize Array(w372, 8 ("维数大小")) -> (w384:string[])
                n326 = Initialize Array(w372, 5 ("维数大小")) -> (w376:string[])
                n327 = Initialize Array(w372, 6 ("维数大小")) -> (w375:string[])
                n328 = Initialize Array(w372, 15 ("维数大小")) -> (w379:string[])
                n329 = Array To Cluster(array=w375) -> (cluster=w374:T13)
                n330 = Array To Cluster(array=w384) -> (cluster=w383:T14)
                n331 = Array To Cluster(array=w376) -> (cluster=w377:T15)
                n332 = global write "全局 时间2.vi" "跨度核查索引"(w383) -> ()
                n333 = global write "全局 时间2.vi" "零点核查索引"(w383) -> ()
                n334 = global write "全局 时间2.vi" "平行样索引"(w377) -> ()
                n335 = global write "全局 时间2.vi" "加标回收索引"(w377) -> ()
                n336 = global write "全局 时间2.vi" "仪器日志索引"(w374) -> ()
                n337 = Array To Cluster(array=w379) -> (cluster=w380:T16)
                n338 = global write "全局 时间2.vi" "标样核查索引"(w380) -> ()
                n339 = global write "全局 时间2.vi" "集成干预索引"(w380) -> ()
              }
              frame True {
              }
            }
            n340 = Initialize Array(w358, 34 ("维数大小")) -> (w367:string[])
            n341 = Initialize Array(w358, 13 ("维数大小")) -> (w363:string[])
            n342 = Initialize Array(w358, 6 ("维数大小")) -> (w361:string[])
            n343 = Array To Cluster(array=w361) -> (cluster=w360:T13)
            n344 = global write "全局 时间2.vi" "仪器日志索引"(w360) -> ()
            n345 = Array To Cluster(array=w367) -> (cluster=w366:T17)
            n346 = Array To Cluster(array=w363) -> (cluster=w364:T18)
            n347 = global write "全局 水样时间.vi" "水样数据索引"(w366) -> ()
            n348 = global write "全局 时间2.vi" "仪器参数索引"(w364) -> ()
          }
        }
      }
      event "开机启动": Value Change {
        n349 = event-data() -> ("CtlRef"=w386:refnum<vi>, "OldVal"=w385:bool, "NewVal"=w387:bool)  [unwired: 1 in, 3 out]
        n350 = case shown="真" w387 {
          tunnel: w386 -> [w389 w402]
          tunnel: w385 -> [w388 w401]
          frame False {
            n351 = Two Button Dialog(message="是否删除开机启动？" ("消息"), 1:"否" ("F按钮名称（“取消”）"), 2:"是" ("T按钮名称（“确定”）")) -> (T button?=w390:bool)
            n352 = case shown="假" w390 {
              tunnel: w389 -> [w395 _]
              tunnel: w388 -> [w394 _]
              frame False {
                n353 = property class="Bool (严格)"(reference=w395, "Value"=w394) -> ()  [unwired: 1 in, 2 out]
              }
              frame True {
                n354 = call <vilib>:"Application Directory.vi"() -> ("Application Directory"=w397:path)
                n355 = call "删除启动项.vi"("启动文件路径"=w397) -> ("删除标记"=w396:bool)  [unwired: 9 in, 1 out]
                n356 = case shown="假" w396 {
                  tunnel: ["删除开机启动失败" ("T按钮名称（“确定”）") "删除开机启动成功" ("T按钮名称（“确定”）")] -> w398
                  frame False {
                  }
                  frame True {
                  }
                }
                n357 = One Button Dialog(message=w398) -> ()  [unwired: 1 in, 1 out]
              }
            }
          }
          frame True {
            n358 = Two Button Dialog(message="是否添加开机启动？" ("消息"), 1:"否" ("F按钮名称（“取消”）"), 2:"是" ("T按钮名称（“确定”）")) -> (T button?=w403:bool)
            n359 = case shown="真" w403 {
              tunnel: w402 -> [w408 _]
              tunnel: w401 -> [w407 _]
              frame False {
                n360 = property class="Bool (严格)"(reference=w408, "Value"=w407) -> ()  [unwired: 1 in, 2 out]
              }
              frame True {
                n361 = call <vilib>:"Application Directory.vi"() -> ("Application Directory"=w411:path)
                n362 = call "添加启动项.vi"("启动文件路径"=w411) -> ("添加成功标记"=w410:bool)  [unwired: 9 in, 1 out]
                n363 = case shown="真" w410 {
                  tunnel: ["添加开机启动失败" ("T按钮名称（“确定”）") "添加开机启动成功" ("T按钮名称（“确定”）")] -> w409
                  frame False {
                  }
                  frame True {
                  }
                }
                n364 = One Button Dialog(message=w409) -> ()  [unwired: 1 in, 1 out]
              }
            }
          }
        }
      }
      event "更新": Value Change {
        n365 = event-data() -> ()  [unwired: 1 in, 6 out]
        n366 = call "自定义双按钮对话框.vi"("消息"="选择是否从服务器获取最新版本信息？") -> ("输出"=w414:bool)  [unwired: 10 in]
        n367 = case shown="真" w414 {
          frame False {
          }
          frame True {
            w422 = T19 2 items=["两端", "字符串首端", "字符串末端"] ("location (both)")
            w418 = "/" ("分隔符(Tab)")
            # "获取最新版本"
            n368 = local read "updateconfiguration"() -> (w431:T1)
            n369 = Unbundle By Name(w431) -> ("主机"=w430:string, "用户"=w419:string, "密码"=w429:string, "远程路径"=w427:string)
            n370 = Spreadsheet String To Array(delimiter (Tab)="\\" ("分隔符(Tab)"), format string="" ("格式字符串"), spreadsheet string=w427, array type (2D Dbl)=string[] []) -> (array=w424:string[])
            n371 = Array To Spreadsheet String(delimiter (Tab)=w418, array=w424, 3:"%s" ("格式字符串")) -> (spreadsheet string=w417:string)
            n372 = Concatenate Strings(w418, w417) -> (w416:string)
            n373 = call <vilib>:"Trim Whitespace.vi"("string"=w416, "location (both)"=w422) -> ("trimmed string"=w421:string)
            n374 = Bundle By Name(cluster=T11 {"host"="27.154.58.30", "port"=8020, "user"="std", "password"="std23506", "远端地址"="/微站/室外总磷总氮高压过滤无主板新电路板/一体化微型水质监测站.exe"} ("服务器信息"), "host"=w430, "port"=u16 8020, "user"=w419, "password"=w429, "远端地址"=w421) -> (w432:T11)
            n375 = call "Update.vi"("服务器信息"=w432) -> ()  [unwired: 11 in]
          }
        }
      }
      event "updateconfiguration": Value Change {
        n376 = event-data() -> ("NewVal"=w441:T1)  [unwired: 1 in, 5 out]
        n377 = call <vilib>:"Application Directory.vi"() -> ("Application Directory"=w445:path)
        n378 = Build Path(base path=w445, name or relative path="update\\data\\set.ini" ("名称或相对路径")) -> (appended path=w443:path)
        n379 = Build Array("主机" ("section"), "用户" ("section"), "密码" ("key"), "远程路径" ("key"), "下载文件名" ("key"), "软件版本" ("key")) -> (w434:string[])
        n380 = call "配置文件write.vi"("updateconfiguration"=w441, "configuration file path"=w443, "键数组"=w434, "段"="应用程序交互" ("section")) -> ("error out"=w442:errorcluster)  [unwired: 7 in]
        n381 = call <vilib>:"Clear Errors.vi"("error in (no error)"=w442) -> ()  [unwired: 5 in, 2 out]
      }
      event "IP", "PORT": Mouse Down {
        n382 = event-data() -> ("CtlRef"=w455:refnum<vi>)  [unwired: 1 in, 7 out]
        n383 = property class="Str"(reference=w455) -> (reference out=w453:refnum<vi>, "Value"=w454:string)  [unwired: 1 in, 1 out]
        n384 = call "IP键盘.vi"("OldNumber"=w454) -> ("NewNumber"=w450:string)
        n385 = String Length(string=w450) -> (length=w452:i32)
        n386 = Less Or Equal?(x=w452, y=15) -> (x <= y?=w449:bool)
        n387 = case shown="假" w449 {
          tunnel: w453 -> [w456 w460]
          tunnel: w450 -> [_ w459]
          tunnel: [w456 w460] -> w448
          tunnel: ["127.0.0.1" w459] -> w447
          frame False {
            n388 = One Button Dialog(message="超过ipv4最大长度限制,请重新输入!" ("消息")) -> ()  [unwired: 1 in, 1 out]
          }
          frame True {
          }
        }
        n389 = property class="Str"(reference=w448, "Val(Sgnl)"=w447) -> ()  [unwired: 1 in, 2 out]
      }
    }
  }
  n390 = while {
    shift-right: [w462] -> _
    shift-left: "数  据  采  集  传  输  系  统" ("标题显示") -> [w463]
    stop <- FALSE stop-if-true
    n391 = call "字符串移位显示.vi"("字符框大小"=72, "字符串输入"=w463) -> ("移位后字符串"=w462:string)  [unwired: 8 in, 1 out]
    "标题显示" <- w462
    n392 = Wait (ms)(milliseconds to wait=u32 1000 ("等待时间（毫秒）")) -> ()  [unwired: 1 out]
  }
